vi "Reset on Start.vi"(8 "error in (no error)":errorcluster, 9 "Outer Loop State":T1 {"Phi Setpoint" format="%#_13g"}) -> (0 "error out":errorcluster, 1 "Phi Setpoint":dbl, 2 "Gamma Setpoint":dbl, 3 "Balance Iteration Counter":dbl)   [LabVIEW 2014]
uses:
  Start.vi
  <userlib>/UCSD Robotics Lab/Robotics-Cape/LV/libroboticscape.lvlib
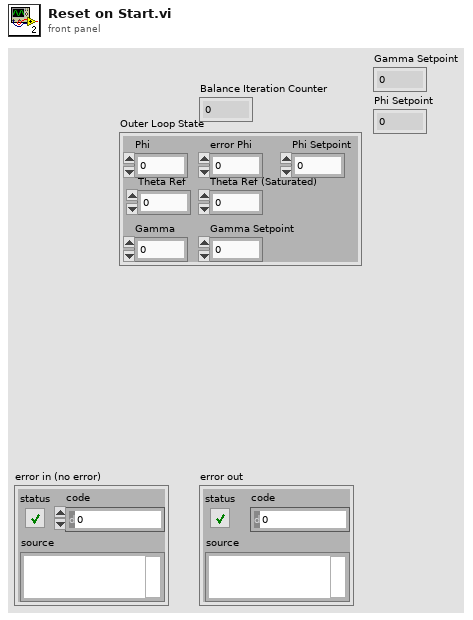
[diagram p1: front panel]
types:
  T1 = cluster{"Phi":dbl, "error Phi":dbl, "Gamma":dbl, "Theta Ref":dbl, "Theta Ref (Saturated)":sgl, "Gamma Setpoint":dbl, "Phi Setpoint":dbl}
  T2 = cluster{"Upright Counter":dbl, "Theta (Deg)":dbl, "Theta (Rad)":dbl, "eTheta":dbl, "U":dbl, "Steering U":dbl, "U saturated":sgl}
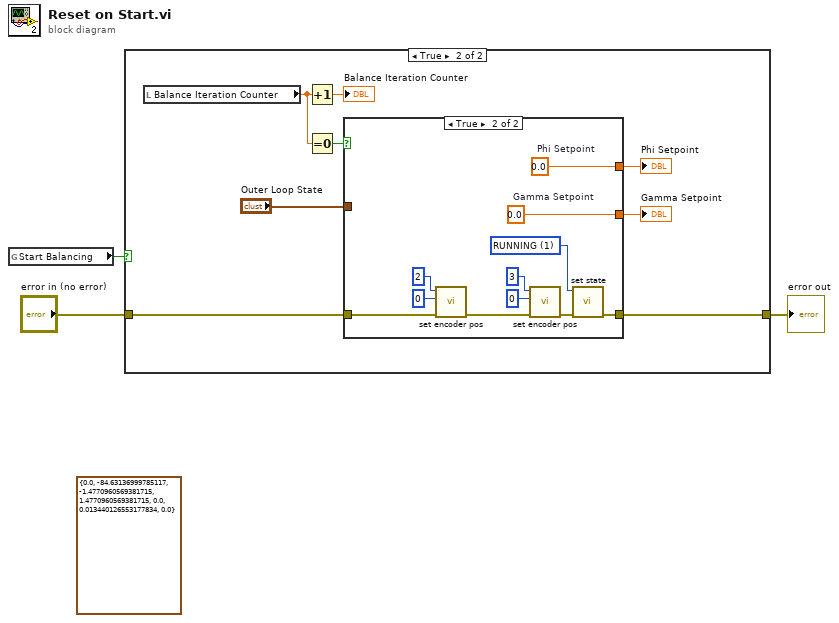
[diagram p0: block diagram]
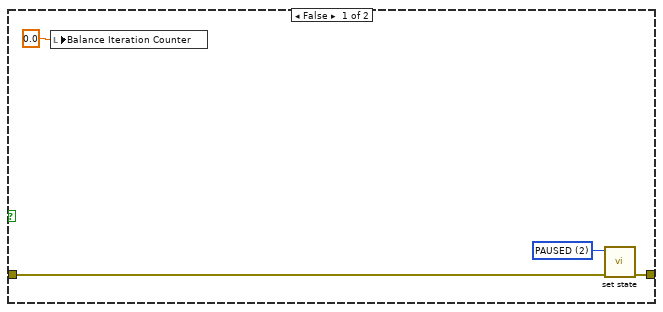
[diagram p2: hidden frame]
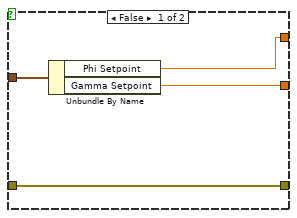
[diagram p3: hidden frame]
diagram:
  (unwired) T2 {"Upright Counter"=0.0, "Theta (Deg)"=-84.63136999785117, "Theta (Rad)"=-1.4770960569381715, "eTheta"=1.4770960569381715, "U"=0.0, "Steering U"=0.013440126553177834, "U saturated"=0.0} ("Inner Loop State")
  n1 = global read "Start.vi" "Start Balancing"() -> (w1:bool)
  n2 = case shown="True" w1 {
    tunnel: "error in (no error)" -> [w6 w15]
    tunnel: [w5 w14] -> w2
    frame False {
      w7 = u32 2 items=["UNINITIALIZED", "RUNNING", "PAUSED", "EXITING"] ("new_state")
      n3 = local write "Balance Iteration Counter"(0.0 ("Balance Iteration Counter")) -> ()
      n4 = call <userlib>:"set state.vi"("error in (no error)"=w6, "new_state"=w7) -> ("error out"=w5:errorcluster)  [unwired: 8 in, 1 out]
    }
    frame True {
      n5 = local read "Balance Iteration Counter"() -> (w11:dbl)
      n6 = Increment(x=w11) -> (x+1=→"Balance Iteration Counter":dbl)
      n7 = Equal To 0?(x=w11) -> (x = 0?=w13:bool)
      n8 = case shown="True" w13 {
        tunnel: w15 -> [w19 w23]
        tunnel: [w19 w29] -> w14
        tunnel: [w16 w21] -> w10
        tunnel: [w17 w20] -> w9
        tunnel: "Outer Loop State" -> [w18 _]
        frame False {
          n9 = Unbundle By Name(w18) -> ("Phi Setpoint"=w17:dbl, "Gamma Setpoint"=w16:dbl)
        }
        frame True {
          w20 = 0.0  # Phi Setpoint
          w21 = 0.0  # Gamma Setpoint
          w30 = u32 1 items=["UNINITIALIZED", "RUNNING", "PAUSED", "EXITING"] ("new_state")
          n10 = call <userlib>:"set encoder pos.vi"("error in (no error)"=w23, "value"=0, "ch"=2) -> ("error out"=w24:errorcluster)  [unwired: 7 in, 1 out]
          n11 = call <userlib>:"set encoder pos.vi"("error in (no error)"=w24, "value"=0, "ch"=3) -> ("error out"=w22:errorcluster)  [unwired: 7 in, 1 out]
          n12 = call <userlib>:"set state.vi"("error in (no error)"=w22, "new_state"=w30) -> ("error out"=w29:errorcluster)  [unwired: 8 in, 1 out]
        }
      }
      "Gamma Setpoint" <- w10
      "Phi Setpoint" <- w9
    }
  }
  "error out" <- w2
